vi "fma.vi"() -> ()   [LabVIEW 2025]
uses:
  ArrayFMAMSVC/FMA/x64/Release/FMA.dll
panel:
  out "x = y?":bool
  out "time, s 2":dbl
  out "sum":sgl
  out "time, s":dbl
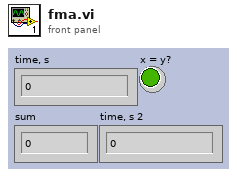
[diagram p1: front panel]
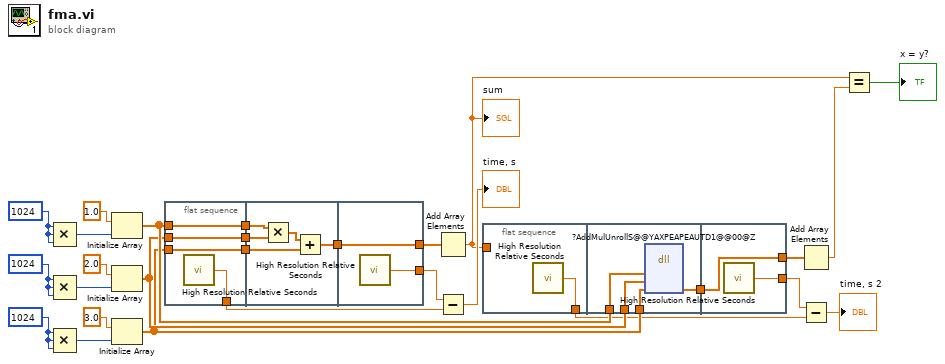
[diagram p0: block diagram]
diagram:
  w20 = 1024
  w23 = 1024
  w26 = 1024
  n1 = Compound Arithmetic op=MULTIPLY(w26, w26, w26) -> (w27:i32)
  n2 = Compound Arithmetic op=MULTIPLY(w23, w23, w23) -> (w24:i32)
  n3 = Compound Arithmetic op=MULTIPLY(w20, w20, w20) -> (w21:i32)
  n4 = Initialize Array(sgl 1.0 ("element"), w27) -> (w11:sgl[])
  n5 = Initialize Array(sgl 2.0 ("element"), w24) -> (w10:sgl[])
  n6 = Initialize Array(sgl 3.0 ("element"), w21) -> (w9:sgl[])
  n7 = flat-sequence {
    tunnel: w9 -> [w30]
    tunnel: w10 -> [w31]
    tunnel: w11 -> [w32]
    tunnel: [w32] -> w18
    tunnel: [w31] -> w17
    tunnel: [w30] -> w16
    tunnel: [w29] -> w14
    tunnel: [w33] -> w19
    tunnel: w18 -> [w37]
    tunnel: w17 -> [w36]
    tunnel: w16 -> [w34]
    tunnel: [w39] -> w12
    tunnel: w19 -> [w39]
    tunnel: [w38] -> w15
    frame #0 {
      n8 = call <vilib>:"High Resolution Relative Seconds.vi"() -> ("relative seconds"=w29:dbl)
    }
    frame #1 {
      n9 = Multiply(x=w37, y=w36) -> (x*y=w35:sgl[])
      n10 = Add(x=w35, y=w34) -> (x+y=w33:sgl[])
    }
    frame #2 {
      n11 = call <vilib>:"High Resolution Relative Seconds.vi"() -> ("relative seconds"=w38:dbl)
    }
  }
  n12 = Add Array Elements(numeric array=w12) -> (sum=w2:sgl)
  "sum" <- w2
  n13 = Subtract(x=w15, y=w14) -> (x-y=→"time, s":dbl)
  n14 = flat-sequence {
    tunnel: [w40] -> w6
    tunnel: w2 -> [_]
    tunnel: w11 -> [w44]
    tunnel: w10 -> [w43]
    tunnel: w9 -> [w42]
    tunnel: [w41] -> w5
    tunnel: [w46] -> w7
    tunnel: [w45] -> w4
    tunnel: w5 -> [w45]
    frame #0 {
      n15 = call <vilib>:"High Resolution Relative Seconds.vi"() -> ("relative seconds"=w40:dbl)
    }
    frame #1 {
      n16 = dll-call lib="C:/Users/Andrey/Desktop/blog/drafts/LV_Memory/FMA/ArrayFMAMSVC/FMA/x64/Release/FMA.dll" fn="?AddMulUnrollS@@YAXPEAPEAUTD1@@00@Z"("a"=w44, "b"=w43, "c"=w42) -> ("c"=w41:sgl[])  [unwired: 6 in, 2 out]
    }
    frame #2 {
      n17 = call <vilib>:"High Resolution Relative Seconds.vi"() -> ("relative seconds"=w46:dbl)
    }
  }
  n18 = Add Array Elements(numeric array=w4) -> (sum=w3:sgl)
  n19 = Subtract(x=w7, y=w6) -> (x-y=→"time, s 2":dbl)
  n20 = Equal?(x=w2, y=w3) -> (x = y?=→"x = y?":bool)
